vi "SerialWindow.vi"() -> ()   [LabVIEW 2020]
uses:
  <vilib>/Instr/_visa.llb/VISA Configure Serial Port (Instr).vi
panel:
  out "Cover":bool
  out "name":string
  in  "Write text":string
  in  "REPL":string
  in  "Connect":bool
  in  "Stop Button":bool
  in  "Port":refnum<visa-resource-name>
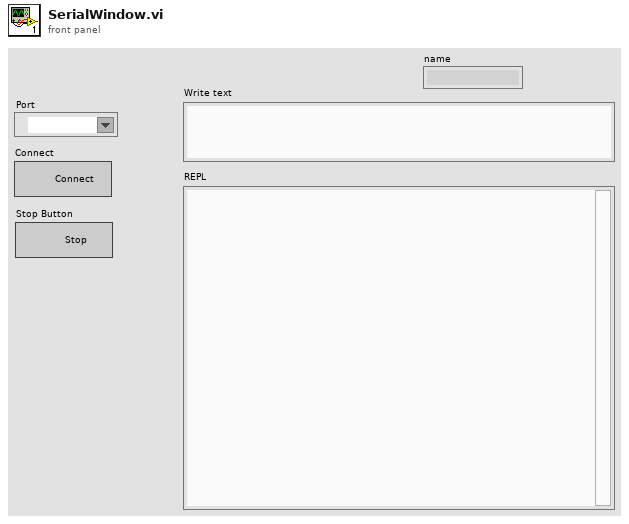
[diagram p1: front panel]
types:
  T1 = cluster{"cmd":string, "path":string, "http ver":string}
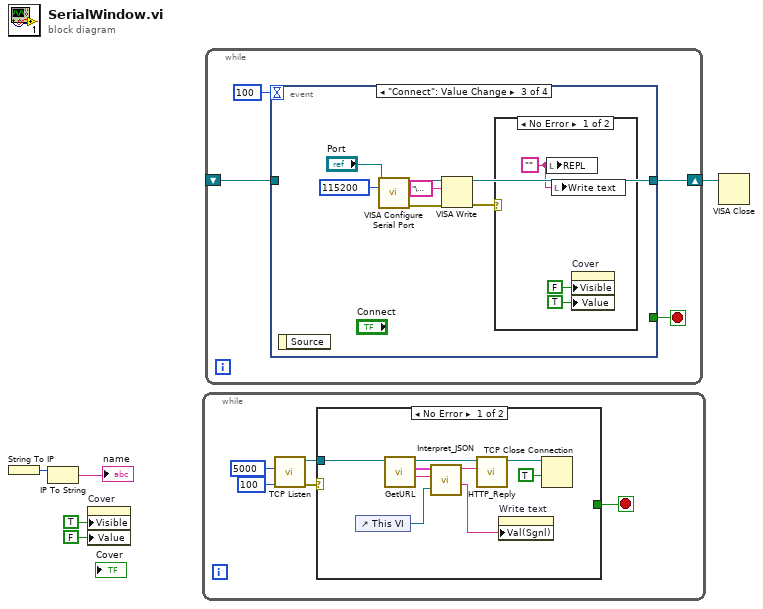
[diagram p0: block diagram]
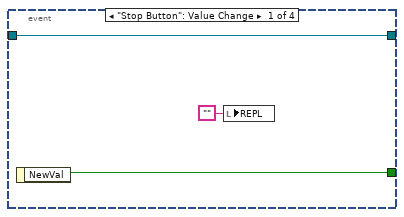
[diagram p2: hidden frame]
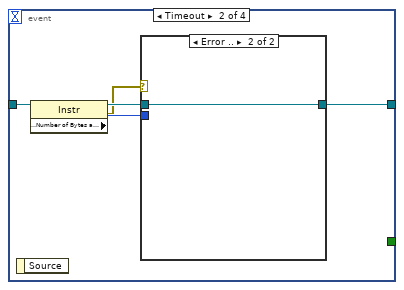
[diagram p3: hidden frame]
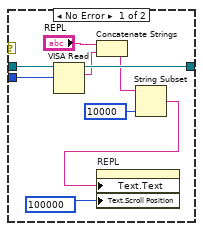
[diagram p4: hidden frame]
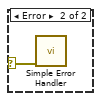
[diagram p5: hidden frame]
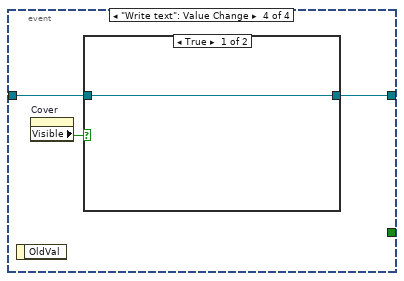
[diagram p6: hidden frame]
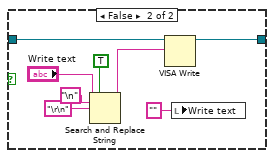
[diagram p7: hidden frame]
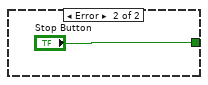
[diagram p8: hidden frame]
diagram:
  n1 = String To IP() -> (0:w5:u32)  [unwired: 1 in]
  n2 = IP To String(2:w5) -> (0:→"name":string)  [unwired: 1 in]
  n3 = property on="Cover" class="Bool (strict)"("Visible"=TRUE, "Value"=FALSE ("Cover")) -> ()  [unwired: 2 in, 2 out]
  n4 = while {
    stop <- w6 stop-if-true
    n5 = call <vilib>:"TCP Listen.vi"("timeout ms (wait forever: -1)"=100, "port"=u16 5000) -> ("error out"=w9:errorcluster, "connection ID"=w8:refnum<k5>)  [unwired: 5 in, 3 out]
    n6 = case shown="No Error" w9 {
      tunnel: w8 -> [w19 _]
      tunnel: [_ "Stop Button"] -> w6
      frame No Error {
        n7 = control-ref of="This VI"() -> (w11:refnum<vi>)
        n8 = call "GetURL.vi"("TCP"=w19) -> ("payload"=w14:string, "path"=w15:T1, "TCP out"=w16:refnum<k5>)  [unwired: 7 in, 1 out]
        n9 = call "Interpret_JSON.vi"("This VI"=w11, "payload"=w14, "path"=w15) -> ("Output"=w12:string, "Reply"=w13:string)  [unwired: 7 in]
        n10 = call "HTTP_Reply.vi"("input in"=w13, "TCP in"=w16) -> ("TCP out"=w18:refnum<k5>)  [unwired: 9 in]
        n11 = property on="Write text" class="Str"("Val(Sgnl)"=w12) -> ()  [unwired: 2 in, 2 out]
        n12 = TCP Close Connection(connection ID=w18, abort (F)=TRUE) -> ()  [unwired: 1 in, 2 out]
      }
      frame Error {
      }
    }
  }
  n13 = while {
    shift-right: [w23] -> w1
    shift-left: _ -> [w22]
    stop <- w24 stop-if-true
    n14 = event shown="[2] \"Connect\": Value Change" {
      selector: _ -> [_ _ _ _]
      dyn-events: _ -> [_ _ _ _]
      timeout: 100 -> [_ _ _ _]
      tunnel: [w25 _ _ _] -> w24
      tunnel: [w26 w30 w45 w54] -> w23
      tunnel: w22 -> [w26 w29 _ w55]
      event "Stop Button": Value Change {
        n15 = event-data() -> ("NewVal"=w25:bool)  [unwired: 1 in]
        n16 = local write "REPL"("") -> ()
      }
      event Timeout {
        n17 = event-data() -> ()  [unwired: 1 in, 1 out]
        n18 = property class="Instr"(reference=w29) -> (error out=w28:errorcluster, "Serial Settings:Number of Bytes at Serial Port"=w31:u32)  [unwired: 1 in, 1 out]
        n19 = case shown="Error .." w28 {
          tunnel: w31 -> [w40 _]
          tunnel: [w39 w41] -> w30
          tunnel: w29 -> [w38 w41]
          frame No Error {
            n20 = VISA Read(VISA resource name=w38, byte count=w40) -> (VISA resource name out=w39:refnum<visa-resource-name>, read buffer=w37:string)  [unwired: 1 in, 2 out]
            n21 = Concatenate Strings("REPL", w37) -> (w36:string)
            n22 = String Subset(string=w36, length (rest)=10000 ("length (rest)")) -> (substring=w32:string)  [unwired: 1 in]
            n23 = property on="REPL" class="Str"("Text.Text"=w32, "Text.Scroll Position"=u32 100000 ("Text.Selection:Start")) -> ()  [unwired: 2 in, 2 out]
          }
          frame Error {
          }
        }
      }
      event "Connect": Value Change {
        n24 = event-data() -> ()  [unwired: 1 in, 1 out]
        n25 = call-poly "VISA Configure Serial Port"("VISA resource name"="Port", "baud rate (9600)"=u32 115200) -> ("VISA resource name out"=w46:refnum<visa-resource-name>, "error out"=w43:errorcluster)  [unwired: 12 in]
        n26 = VISA Write(VISA resource name=w46, write buffer="\u0003", error in (no error)=w43) -> (VISA resource name out=w45:refnum<visa-resource-name>, error out=w42:errorcluster)  [unwired: 1 out]
        n27 = case shown="No Error" w42 {
          selector: w42 -> [_ w52]
          frame No Error {
            w51 = ""
            n28 = local write "REPL"(w51) -> ()
            n29 = local write "Write text"(w51) -> ()
            n30 = property on="Cover" class="Bool (strict)"("Visible"=FALSE, "Value"=TRUE ("Cover")) -> ()  [unwired: 2 in, 2 out]
          }
          frame Error {
            n31 = call <vilib>:"Simple Error Handler.vi"("error in (no error)"=w52) -> ()  [unwired: 4 in, 5 out]
          }
        }
      }
      event "Write text": Value Change {
        n32 = event-data() -> ()  [unwired: 1 in, 1 out]
        n33 = property on="Cover" class="Bool (strict)"() -> ("Visible"=w53:bool)  [unwired: 2 in, 2 out]
        n34 = case shown="True" w53 {
          tunnel: w55 -> [w56 w64]
          tunnel: [w56 w63] -> w54
          frame True {
          }
          frame False {
            n35 = Search and Replace String(replace all?=TRUE ("replace all? (F)"), input string="Write text", search string="\n" ("input string"), replace string="\r\n" ("replace string (\"\")")) -> (result string=w59:string)  [unwired: 4 in, 3 out]
            n36 = VISA Write(VISA resource name=w64, write buffer=w59) -> (VISA resource name out=w63:refnum<visa-resource-name>)  [unwired: 1 in, 2 out]
            n37 = local write "Write text"("" ("Write text")) -> ()
          }
        }
      }
    }
  }
  n38 = VISA Close(VISA resource name=w1) -> ()  [unwired: 1 in, 1 out]
